vi "Read ini file.vi"(8 "Error In":errorcluster, 11 "WS1040.lvclass":refnum<class "WS1040.lvclass">) -> (0 "Error Out":errorcluster, 3 "WS1040.lvclass Out":refnum<class "WS1040.lvclass">)   [LabVIEW 2020, in "WS1040.lvclass"]
uses:
  WS1040.lvclass
  Controls/Capacitor register.ctl
  <vilib>/Utility/config.llb/Read Key (Double).vi
  <vilib>/Utility/config.llb/NI_LVConfig.lvlib
  Toggle 6.lvclass
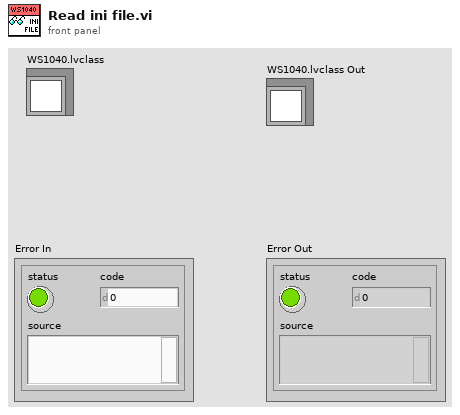
[diagram p1: front panel]
types:
  T1 = typedef "Toggle 6.lvclass/Capacitor register.ctl" = cluster{"Register":u32, "Beam":dbl, "Trimmer":dbl}
  T2 = typedef "NI_LVConfig.lvlib/Config Data RefNum.ctl" = refnum<k1>
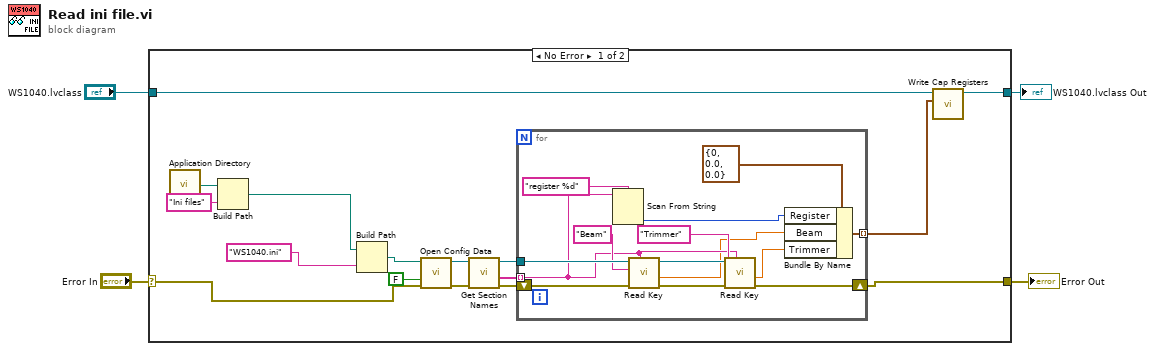
[diagram p0: block diagram]
diagram:
  n1 = case shown="No Error" "Error In" {
    selector: "Error In" -> [w17 w36]
    tunnel: [w10 w36] -> w3
    tunnel: "WS1040.lvclass" -> [w9 w35]
    tunnel: [w8 w35] -> w1
    frame No Error {
      n2 = call <vilib>:"Application Directory.vi"() -> ("Application Directory"=w20:path)
      n3 = Build Path(base path=w20, name or relative path="Ini files") -> (appended path=w6:path)
      n4 = Build Path(base path=w6, name or relative path="WS1040.ini") -> (appended path=w18:path)
      n5 = call <vilib>:"Open Config Data.vi"("error in (no error)"=w17, "create file if necessary (T)"=FALSE, "configuration file path"=w18) -> ("error out"=w15:errorcluster, "refnum"=w14:T2)  [unwired: 6 in, 1 out]
      n6 = call <vilib>:"Get Section Names.vi"("error in (no error)"=w15, "refnum"=w14) -> ("error out"=w13:errorcluster, "section names"=w12:string[], "refnum out"=w11:T2)  [unwired: 7 in]
      n7 = for {
        tunnel: w12 -> [w27] mode=indexing
        tunnel: w11 -> [w33]
        shift-right: [w28] -> w10
        shift-left: w13 -> [w34]
        tunnel: [w21] -> w7 mode=indexing
        n8 = Scan From String(format string="register %d", input string=w27) -> (output 1=w24:i32)  [unwired: 3 in, 3 out]
        n9 = call-poly <vilib>:"Read Key.vi"("section"=w27, "error in (no error)"=w34, "key"="Beam", "refnum"=w33) -> ("error out"=w29:errorcluster, "value"=w23:dbl, "refnum out"=w31:T2)  [unwired: 4 in, 1 out]
        n10 = call-poly <vilib>:"Read Key.vi"("section"=w27, "error in (no error)"=w29, "key"="Trimmer", "refnum"=w31) -> ("error out"=w28:errorcluster, "value"=w22:dbl)  [unwired: 4 in, 2 out]
        n11 = Bundle By Name(cluster=T1 {"Register"=0, "Beam"=0.0, "Trimmer"=0.0} ("Cap register"), "Register"=w24, "Beam"=w23, "Trimmer"=w22) -> (w21:T1)
      }
      n12 = call-dynamic "Write Cap Registers.vi"("Cap Registers"=w7, "Toggle 6 in"=w9) -> ("Toggle 6 out"=w8:refnum<class "WS1040.lvclass">)  [unwired: 9 in]
    }
    frame Error {
    }
  }
  "Error Out" <- w3
  "WS1040.lvclass Out" <- w1
